vi "MCL Get Firmware Version.vi"(9 "handle":i32, 10 "profile":i16, 11 "version":i16) -> (1 "function return":i32, 2 "profile out":i16, 3 "version out":i16)   [LabVIEW 2017, in "Madlib.lvlib"]
doc: "MADLIB_API int MCL_GetFirmwareVersion(short *version, short *profile, int handle);"
uses:
  Madlib.lvlib
  Madlib.dll
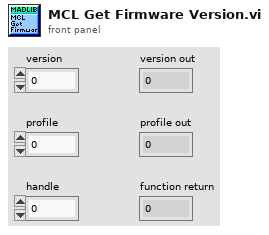
[diagram p1: front panel]
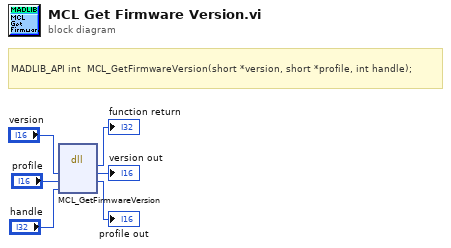
[diagram p0: block diagram]
diagram:
  # "MADLIB_API\tint \tMCL_GetFirmwareVersion(short *version, short *profile, int handle);"
  n1 = dll-call lib="C:/Users/francesco/dev/pump-probe/Piezo/lvlib/Madlib.*" fn="MCL_GetFirmwareVersion"("version"="version", "profile"="profile", "handle"="handle") -> (→"function return":i32, "version"=→"version out":i16, "profile"=→"profile out":i16)  [unwired: 4 in, 2 out]
